vi "Print.vi"(11 "Time Stamp in":refnum<class "Time Stamp.lvclass">) -> (2 "Time Stamp":string, 3 "Time Stamp out":refnum<class "Time Stamp.lvclass">)   [LabVIEW 2023, in "HAL.lvlib" / "Time Stamp.lvclass"]
uses:
  Time Stamp.lvclass
  Time Stamp.lvclass/Time Stamp.ctl
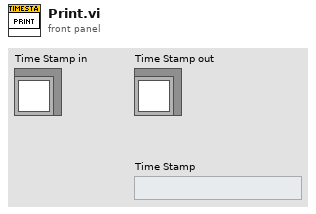
[diagram p1: front panel]
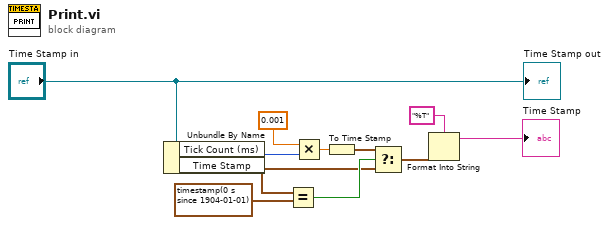
[diagram p0: block diagram]
diagram:
  n1 = Unbundle By Name("Time Stamp in") -> ("Tick Count (ms)"=w9:u64, "Time Stamp"=w4:timestamp)
  n2 = Equal?(x=w4, y=timestamp(0 s since 1904-01-01)) -> (x = y?=w8:bool)
  n3 = Multiply(x=0.001, y=w9) -> (x*y=w6:dbl)
  n4 = To Time Stamp(1:w6) -> (0:w7:timestamp)
  n5 = Select(t=w7, s=w8, f=w4) -> (s? t:f=w3:timestamp)
  n6 = Format Into String(format string="%T", w3) -> (resulting string=→"Time Stamp":string)  [unwired: 2 in, 1 out]
  "Time Stamp out" <- "Time Stamp in"
